vi "choosePath.vi"(8 "error in (no error)":errorcluster, 11 "Pixelfly in":refnum<class "PixelflySA.lvclass">) -> (0 "error out":errorcluster, 2 "Path":path, 3 "Pixelfly out":refnum<class "PixelflySA.lvclass">)   [LabVIEW 2009, in "PixelflySA.lvclass"]
uses:
  PixelflySA.lvclass
  PixelflySA.lvclass/PixelflySA.ctl
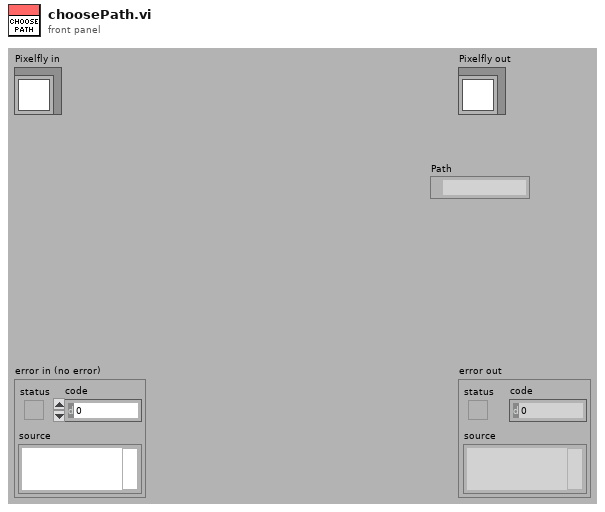
[diagram p1: front panel]
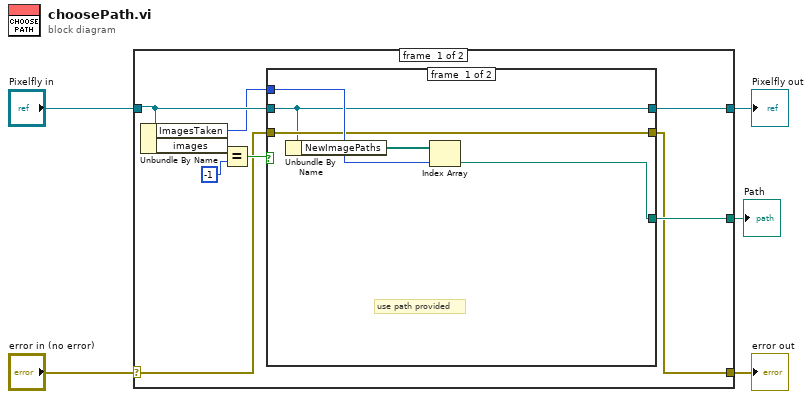
[diagram p0: block diagram]
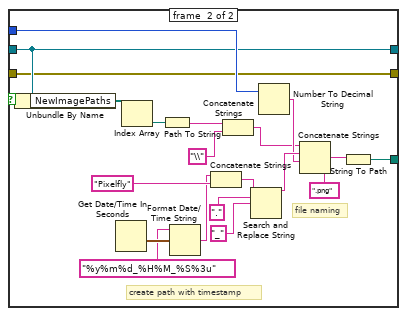
[diagram p2: hidden frame]
diagram:
  n1 = case shown="No Error" "error in (no error)" {
    selector: "error in (no error)" -> [w9 w41]
    tunnel: [w6 w41] -> w4
    tunnel: [w13 w40] -> w2
    tunnel: "Pixelfly in" -> [w14 w40]
    tunnel: [w7 _] -> w1
    frame #0 {
      n2 = Unbundle By Name(w14) -> ("ImagesTaken"=w8:i32, "images"=w12:i32)
      n3 = Equal?(x=w12, y=-1) -> (x = y?=w10:bool)
      n4 = case shown="False" w10 {
        tunnel: w14 -> [w15 w21]
        tunnel: [w15 w21] -> w13
        tunnel: w9 -> [w16 w20]
        tunnel: w8 -> [w19 w27]
        tunnel: [w16 w20] -> w6
        tunnel: [w18 w25] -> w7
        frame #0 {
          # "use path provided"
          n5 = Unbundle By Name(w15) -> ("NewImagePaths"=w17:path[])
          n6 = Index Array(array=w17, index=w19) -> (element=w18:path)
        }
        frame #1 {
          # "create path with timestamp"
          # "file naming"
          n7 = Unbundle By Name(w21) -> ("NewImagePaths"=w22:path[])
          n8 = Get Date/Time In Seconds() -> (seconds since 1Jan1904=w38:timestamp)
          n9 = Index Array(array=w22) -> (element=w23:path)  [unwired: 1 in]
          n10 = Path To String(path=w23) -> (string=w24:string)
          n11 = Format Date/Time String(time format string (%c)="%y%m%d_%H%M_%S%3u", seconds (now)=w38) -> (date/time string=w36:string)  [unwired: 1 in]
          n12 = Concatenate Strings(w36, "Pixelfly") -> (w35:string)
          n13 = Concatenate Strings(w24, "\\") -> (w28:string)
          n14 = Search and Replace String(input string=w35, search string=".", replace string="_") -> (result string=w31:string)  [unwired: 5 in, 3 out]
          n15 = Number To Decimal String(number=w27) -> (decimal integer string=w30:string)  [unwired: 1 in]
          n16 = Concatenate Strings(w28, w31, w30, ".png") -> (w26:string)
          n17 = String To Path(string=w26) -> (path=w25:path)
        }
      }
    }
    frame #1 {
    }
  }
  "error out" <- w4
  "Pixelfly out" <- w2
  "Path" <- w1
